vi "Time.vi"() -> ()   [LabVIEW 2011]
panel:
  out "Waveform Graph":i64[][](graph)
  in  "stop":bool
  out "xml time":timestamp
  out "xml string":string
  out "sbrio time":timestamp
  out "x = y?":bool
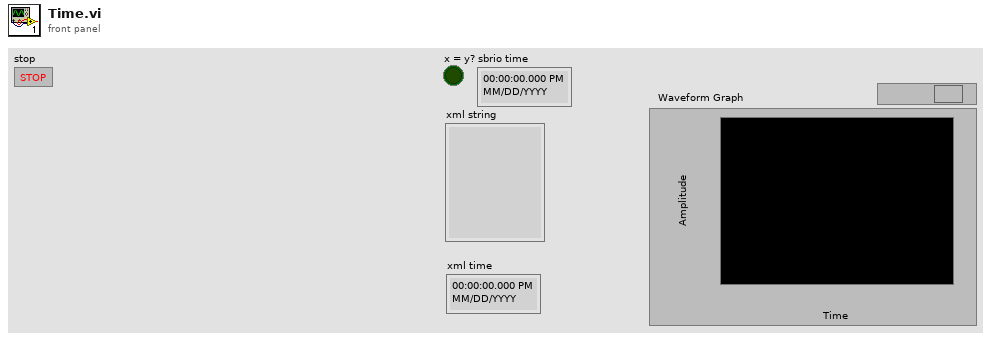
[diagram p1: front panel]
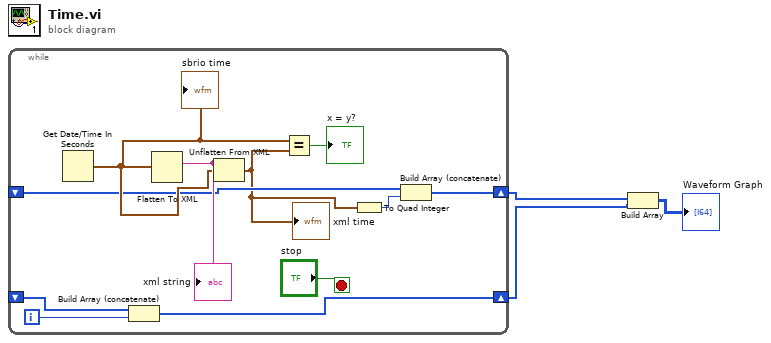
[diagram p0: block diagram]
diagram:
  n1 = while {
    shift-right: [w9] -> w2
    shift-left: _ -> [w8]
    shift-right: [w7] -> w3
    shift-left: _ -> [w6]
    i -> [w10]
    stop <- "stop" stop-if-true
    n2 = Get Date/Time In Seconds() -> (seconds since 1Jan1904=w13:timestamp)
    "sbrio time" <- w13
    n3 = Build Array (concatenate)(w8, w10) -> (w9:i32[])
    n4 = Flatten To XML(anything=w13) -> (xml string=w14:string)
    "xml string" <- w14
    n5 = Unflatten From XML(xml string=w14, type=w13) -> (value=w4:timestamp)  [unwired: 1 in, 1 out]
    "xml time" <- w4
    n6 = Equal?(x=w13, y=w4) -> (x = y?=→"x = y?":bool)
    n7 = To Quad Integer(1:w4) -> (0:w5:i64)
    n8 = Build Array (concatenate)(w6, w5) -> (w7:i64[])
  }
  n9 = Build Array(w3, w2) -> (→"Waveform Graph":i64[][])
